vi "Main.vi"() -> ()   [LabVIEW 2016]
doc: "The roboRIO Project template acquires acceleration data from the onboard accelerometer and displays the changes of acceleration values in a waveform chart."
panel:
  out "To send":i32
  in  "millisecond multiple":u32
  out "Status":u16
  out "Read Status":bool[](array[boolean])
  out "SW4 L":bool
  out "SW4 H":bool
  out "SW3 L":bool
  out "SW3 H":bool
  out "SW2 L":bool
  out "SW2 H":bool
  out "SW1 L":bool
  out "SW1 H":bool
  out "Pot 2":u16
  out "Pot 1":u16
  out "FIFO notEmpty":bool
  in  "stop":bool
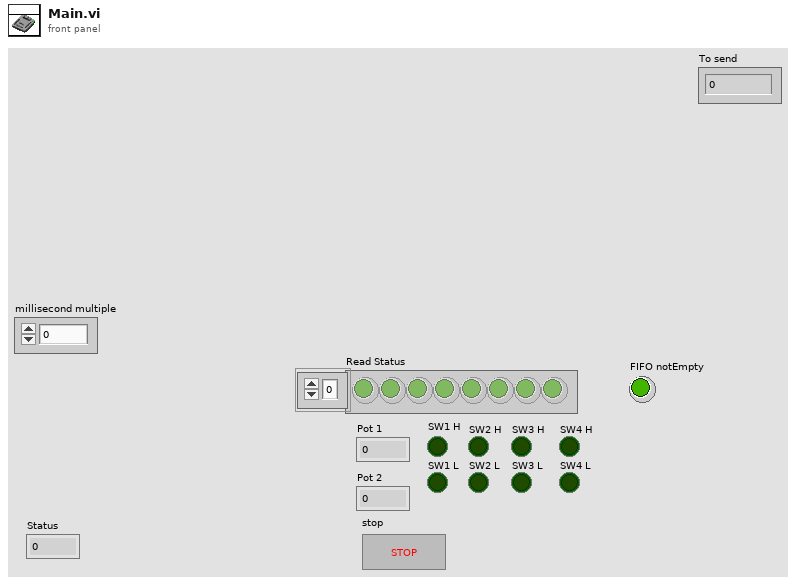
[diagram p1: front panel]
types:
  T1 = typedef "Semaphore RefNum" = refnum<k1>
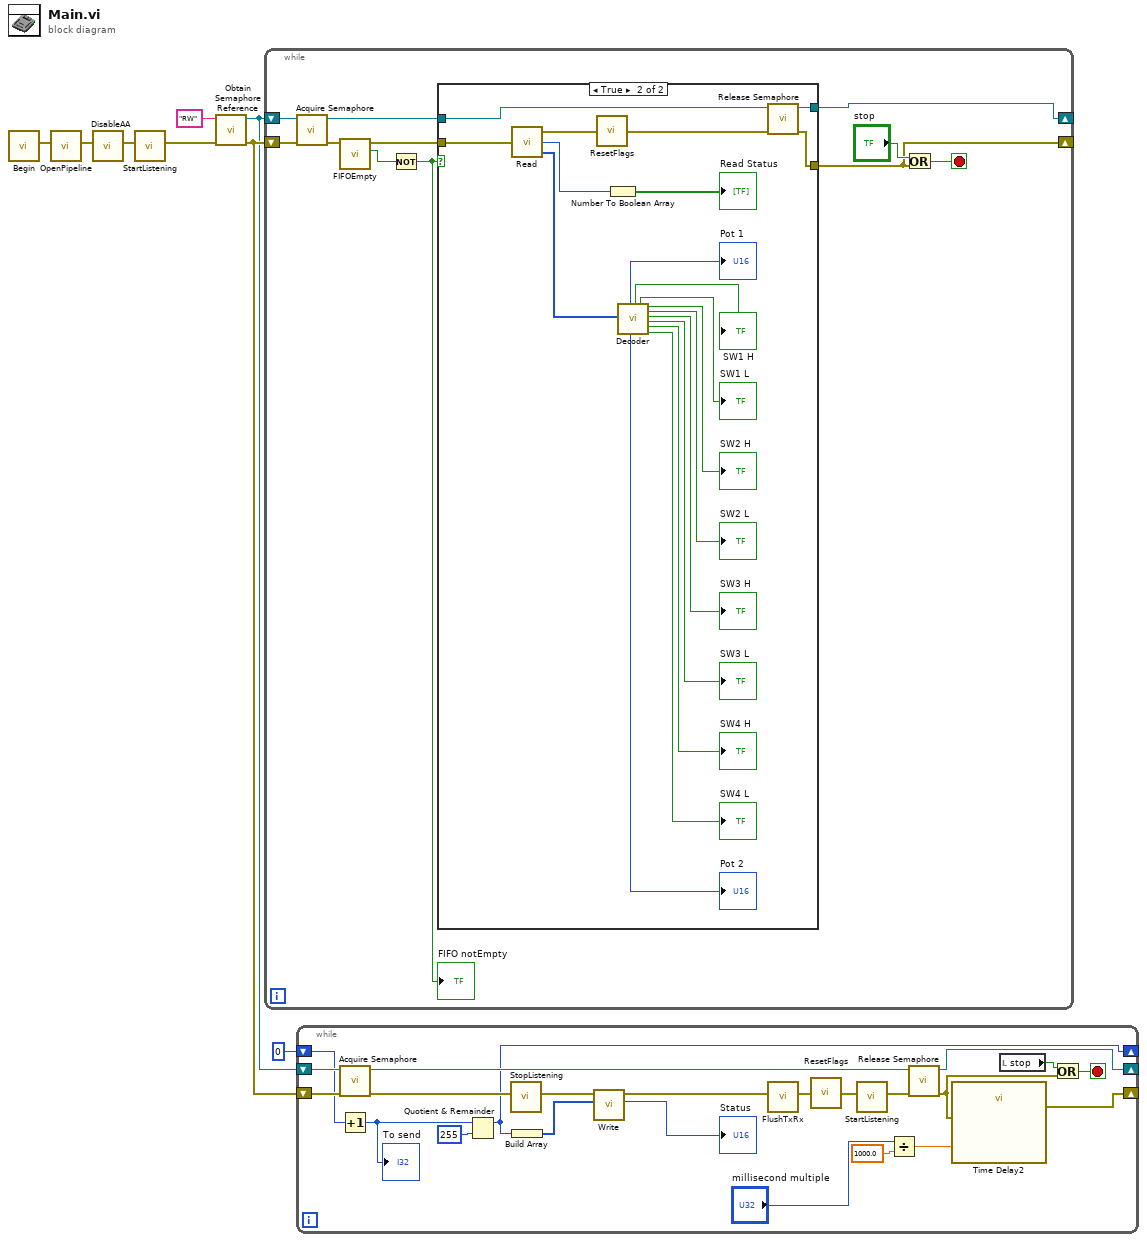
[diagram p0: block diagram]
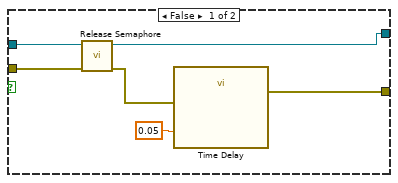
[diagram p2: hidden frame]
diagram:
  n1 = call "Begin.vi"() -> ("error out"=w8:errorcluster)  [unwired: 11 in]
  n2 = call "OpenPipeline.vi"("error in (no error)"=w8) -> ("error out"=w7:errorcluster)  [unwired: 10 in]
  n3 = call "DisableAA.vi"("error in (no error)"=w7) -> ("error out"=w6:errorcluster)  [unwired: 10 in]
  n4 = call "StartListening.vi"("error in (no error)"=w6) -> ("error out"=w5:errorcluster)  [unwired: 10 in]
  n5 = call <vilib>:"Obtain Semaphore Reference.vi"("error in (no error)"=w5, "name (unnamed)"="RW") -> ("error out"=w4:errorcluster, "semaphore"=w2:T1)  [unwired: 3 in, 1 out]
  n6 = while {
    shift-right: [w11] -> _
    shift-left: w4 -> [w13]
    shift-right: [w10] -> _
    shift-left: w2 -> [w14]
    stop <- w18 stop-if-true
    n7 = call <vilib>:"Acquire Semaphore.vi"("error in (no error)"=w13, "semaphore"=w14) -> ("error out"=w12:errorcluster, "semaphore out"=w9:T1)  [unwired: 3 in, 1 out]
    n8 = call "FIFOEmpty.vi"("error in (no error)"=w12) -> ("RX_EMPTY"=w15:bool, "error out"=w19:errorcluster)  [unwired: 9 in]
    n9 = Not(x=w15) -> (.not. x?=w16:bool)
    "FIFO notEmpty" <- w16
    n10 = case shown="True" w16 {
      tunnel: w19 -> [w23 w30]
      tunnel: [w25 w28] -> w11
      tunnel: [w21 w27] -> w10
      tunnel: w9 -> [w22 w26]
      frame False {
        n11 = call <vilib>:"Release Semaphore.vi"("error in (no error)"=w23, "semaphore"=w22) -> ("error out"=w20:errorcluster, "semaphore out"=w21:T1)  [unwired: 4 in]
        n12 = call "Time Delay"("error in (no error)"=w20, "Delay Time (s)"=0.05) -> ("error out"=w25:errorcluster)  [unwired: 9 in]
      }
      frame True {
        n13 = call "Read.vi"("error in (no error)"=w30) -> ("error out"=w44:errorcluster, "Status"=w32:u16, "Data frame"=w43:u16[])
        n14 = call "ResetFlags.vi"("error in (no error)"=w44) -> ("error out"=w29:errorcluster)
        n15 = Number To Boolean Array(number=w32) -> (Boolean array=→"Read Status":bool[])
        n16 = call "Decoder.vi"("Data frame"=w43) -> ("Pot 1"=→"Pot 1":u16, "Pot 2"=→"Pot 2":u16, "SW1 H"=→"SW1 H":bool, "SW1 L"=→"SW1 L":bool, "SW2 H"=→"SW2 H":bool, "SW2 L"=→"SW2 L":bool, "SW3 H"=→"SW3 H":bool, "SW3 L"=→"SW3 L":bool, "SW4 H"=→"SW4 H":bool, "SW4 L"=→"SW4 L":bool)  [unwired: 9 in]
        n17 = call <vilib>:"Release Semaphore.vi"("error in (no error)"=w29, "semaphore"=w26) -> ("error out"=w28:errorcluster, "semaphore out"=w27:T1)  [unwired: 4 in]
      }
    }
    n18 = Or(x="stop", y=w11) -> (x .or. y?=w18:bool)
  }
  n19 = while {
    shift-right: [w49] -> _
    shift-left: w4 -> [w60]
    shift-right: [w55] -> _
    shift-left: w2 -> [w57]
    shift-right: [w45] -> _
    shift-left: 0 -> [w54]
    stop <- w62 stop-if-true
    n20 = call <vilib>:"Acquire Semaphore.vi"("error in (no error)"=w60, "semaphore"=w57) -> ("error out"=w59:errorcluster, "semaphore out"=w56:T1)  [unwired: 3 in, 1 out]
    n21 = Increment(x=w54) -> (x+1=w47:i32)
    "To send" <- w47
    n22 = Quotient & Remainder(x=w47, y=255) -> (x-y*floor(x/y)=w45:i32)  [unwired: 1 out]
    n23 = call "StopListening.vi"("error in (no error)"=w59) -> ("error out"=w67:errorcluster)  [unwired: 10 in]
    n24 = Build Array(w45) -> (w53:i32[])
    n25 = call "Write.vi"("array"=w53, "error in (no error)"=w67) -> ("Status"=→"Status":u16, "error out"=w66:errorcluster)  [unwired: 8 in]
    n26 = call "FlushTxRx.vi"("error in (no error)"=w66) -> ("error out"=w64:errorcluster)  [unwired: 10 in]
    n27 = call "ResetFlags.vi"("error in (no error)"=w64) -> ("error out"=w65:errorcluster)
    n28 = call "StartListening.vi"("error in (no error)"=w65) -> ("error out"=w58:errorcluster)  [unwired: 10 in]
    n29 = Divide(x="millisecond multiple", y=1000.0) -> (x/y=w48:dbl)
    n30 = call <vilib>:"Release Semaphore.vi"("error in (no error)"=w58, "semaphore"=w56) -> ("error out"=w50:errorcluster, "semaphore out"=w55:T1)  [unwired: 4 in]
    n31 = call "Time Delay2"("error in (no error)"=w50, "Delay Time (s)"=w48) -> ("error out"=w49:errorcluster)  [unwired: 9 in]
    n32 = local read "stop"() -> (w61:bool)
    n33 = Or(x=w61, y=w50) -> (x .or. y?=w62:bool)
  }
